vi "Add RT to BC Message.vi"(4 "create timestamp channel":bool, 6 "parameters":T3(array[cluster]), 7 "number of words":u16=1, 8 "error in":errorcluster, 9 "Tx remote terminal":T4, 10 "name":string, 11 "port in":T1 format="%.0x") -> (0 "error out":errorcluster, 1 "BC message":T1=18446744073709551615 format="%.0x", 2 "RT message":T1=18446744073709551615 format="%.0x", 3 "port out":T1 format="%.0x")   [LabVIEW 2020, in "Ballard MIL-STD-1553 Scripting.lvlib"]
uses:
  Ballard MIL-STD-1553 Scripting.lvlib
  <vilib>/NI VeriStand/Custom Device API/Custom Device Item Ref.ctl
  Shared/Terminal Endpoint.ctl
  Shared/Address.ctl
  Shared/Parameter Definition.ctl
  Shared/Message Type.ctl
  <vilib>/NI VeriStand/Custom Device API/Custom Device API.lvlib
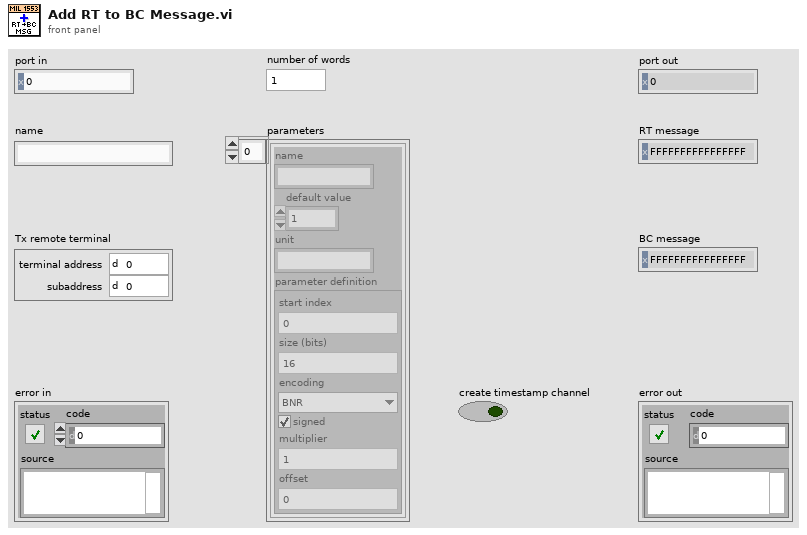
[diagram p1: front panel]
types:
  T1 = typedef "Custom Device API.lvlib/Custom Device Item Ref.ctl" = u64
  T2 = typedef "Parameter Definition.ctl" = cluster{"start index":i32, "size (bits)":i32, "encoding":enum16{"BNR", "BCD", "Discrete"}, "signed":bool, "multiplier":dbl, "offset":dbl}
  T3 = cluster{"name":string, "default value":dbl, "unit":string, "parameter definition":T2}[]
  T4 = typedef "Terminal Endpoint.ctl" = cluster{"terminal address":T5, "subaddress":T5}
  T5 = typedef "Address.ctl" = u16
  T6 = typedef "Message Type.ctl" = string
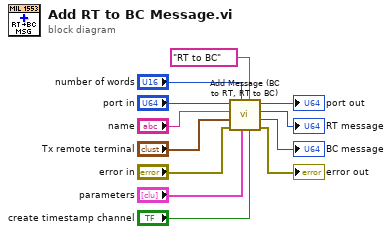
[diagram p0: block diagram]
diagram:
  n1 = call "Add Message (BC to RT, RT to BC).vi"("create timestamp channel"="create timestamp channel", "message type"=T6 "RT to BC", "parameters"="parameters", "number of words"="number of words", "error in"="error in", "remote terminal"="Tx remote terminal", "name"="name", "port in"="port in") -> ("error out"=→"error out":errorcluster, "BC message"=→"BC message":T1, "RT message"=→"RT message":T1, "port out"=→"port out":T1)
